vi "Day 7.vi"() -> ()   [LabVIEW 2023]
panel:
  out "Answer 2":i32
  out "Answer 1":i32
  out "used space":i32
  out "free space":i32
  out "sizes":i32[](array[numeric])
  out "paths":string[](array[string])
  in  "test":bool
  in  "test input":string="$ cd /\n$ ls\ndir a\n14848514 b.txt\n8504156 c.dat\ndir d\n$ cd a\n$ ls\ndir e\n29116 f\n2557 g\n62596 h.lst\n$ cd e\n$ ls\n584 i\n$ cd ..\n$ cd ..\n$ cd d\n$ ls\n4060174 j\n8033020 d.log\n5626152 d.ext\n7214296 k"
  in  "input":string="$ cd /\n$ ls\ndir csjncqmr\ndir fnfjhvsp\ndir mhfrct\ndir pgmgbfcl\ndir qcf\ndir wrsjr\n$ cd csjncqmr\n$ ls\n8827 vdrdm.pfj\n$ cd ..\n$ cd fnfjhvsp\n$ ls\ndir csjncqmr\ndir czpmg\n162385 dcgph\n7135 hff.cdt\n$ cd csjncqmr\n$ ls\n121543 gzjdsn.wlc\ndir ljq\n$ cd ljq\n$ ls\ndir cwlrlvf\ndir jpqjhhpg\n$ cd cwlrlvf\n$ ls\n151219 dcgph\n$ cd ..\n$ cd jpqjhhpg\n$ ls\n188355 dcgph\n38458 gfgl.hlg\n$ cd ..\n$ cd ..\n$ cd ..\n$ cd czpmg\n$ ls\n168232 dcgph\n143031 gzjdsn.wlc\n$ cd ..\n$ cd ..\n$ cd mhfrct\n$ ls\ndir clm\n66710 dcgph\n232576 mtfhpcnj\n$ cd clm\n$ ls\ndir pgmgbfcl\n$ cd pgmgbfcl\n$ ls\n110296 qbfhj.tmn\n$ cd ..\n$ cd ..\n$ cd ..\n$ cd pgmgbfcl\n$ ls\n163613 cgchl\ndir nnlr\n123977 rrwbnmlh.jtt\ndir tjhzggs\ndir wfl\n252837 wpgrl\n$ cd nnlr\n$ ls\n103051 flp\ndir qrhlzd\ndir rcgmhz\ndir snwrlr\ndir vgj\ndir znbzt\n$ cd qrhlzd\n$ ls\ndir crg\n246915 dcgph\n264791 fcphzfb.fmb\n299291 flp\ndir mjqsg\n297202 pgmgbfcl\ndir sbbzgbz\ndir wnsnssbg\n$ cd crg\n$ ls\n55556 flp\n185529 jswdvn\n$ cd ..\n$ cd mjqsg\n$ ls\ndir fnfjhvsp\ndir jfbzjz\ndir rwg\n$ cd fnfjhvsp\n$ ls\n24945 cctwbs\n170960 csjncqmr\n316168 ljffgvvz.zld\n187325 pgmgbfcl.fzv\n74133 qbfhj.tmn\ndir tjhzggs\ndir vjmgmdz\n$ cd tjhzggs\n$ ls\n287777 csjncqmr.nbd\n$ cd ..\n$ cd vjmgmdz\n$ ls\ndir vgpb\n$ cd vgpb\n$ ls\n202578 bbbg.hlr\n$ cd ..\n$ cd ..\n$ cd ..\n$ cd jfbzjz\n$ ls\n207736 tjhzggs.cql\n$ cd ..\n$ cd rwg\n$ ls\n184997 csjncqmr\n4378 dcgph\n55767 qnc.wvv\n$ cd ..\n$ cd ..\n$ cd sbbzgbz\n$ ls\n321376 csjncqmr\n317438 flp\n9263 hrs\n$ cd ..\n$ cd wnsnssbg\n$ ls\ndir jdjv\n$ cd jdjv\n$ ls\n153354 gzjdsn.wlc\n$ cd ..\n$ cd ..\n$ cd ..\n$ cd rcgmhz\n$ ls\ndir tjhzggs\n$ cd tjhzggs\n$ ls\n299192 jfbzjz.ttg\n$ cd ..\n$ cd ..\n$ cd snwrlr\n$ ls\n30314 csjncqmr.jvn\ndir hcf\n$ cd hcf\n$ ls\n81979 jfbzjz.pfz\n179459 ngh\n$ cd ..\n$ cd ..\n$ cd vgj\n$ ls\n278579 jbn.rgz\ndir jzj\ndir lnbhh\ndir pgmgbfcl\ndir qgvspcpm\n$ cd jzj\n$ ls\n295808 hrs\n220437 vqbcl\n$ cd ..\n$ cd lnbhh\n$ ls\n212203 nfmhd.hbq\n233853 qgz.mcd\n$ cd ..\n$ cd pgmgbfcl\n$ ls\ndir mmbdpj\n138462 mwcdrpm.spr\n288430 pgmgbfcl.pwd\n132880 rdmwtn.qjj\n41775 rfqb.djh\ndir rnd\n69597 thnbf\n$ cd mmbdpj\n$ ls\n158542 hrs\n306559 tjhzggs\n$ cd ..\n$ cd rnd\n$ ls\n223745 fnfjhvsp.hgt\n138236 gdmtnffs.cdm\ndir gmzb\ndir hvl\n266178 mzwmjl.rqq\ndir njpq\n33906 qbfhj.tmn\ndir tjhzggs\n$ cd gmzb\n$ ls\n186579 nsbfn.lsd\n$ cd ..\n$ cd hvl\n$ ls\n312925 csjncqmr.sbc\n75264 gqp\n81003 gzjdsn.wlc\n$ cd ..\n$ cd njpq\n$ ls\n188139 lbnrr.pwd\n213545 qgqddvwf.hfl\n$ cd ..\n$ cd tjhzggs\n$ ls\ndir dlwvc\n191782 jfbzjz\ndir tbldpln\n$ cd dlwvc\n$ ls\n75927 jvhjtnft\n260563 qbfhj.tmn\ndir vlg\n$ cd vlg\n$ ls\n187660 hgm\ndir rhr\n273019 tdgr.crr\n$ cd rhr\n$ ls\n286129 wnn.jgn\n$ cd ..\n$ cd ..\n$ cd ..\n$ cd tbldpln\n$ ls\n173546 pdfrsq.pnb\n$ cd ..\n$ cd ..\n$ cd ..\n$ cd ..\n$ cd qgvspcpm\n$ ls\ndir dhrbsl\n286566 fldhvbq\n209725 gzjdsn.wlc\n148148 nspz.gwc\n111003 tjhzggs\n$ cd dhrbsl\n$ ls\n58390 gzjdsn.wlc\n150545 hrs\n$ cd ..\n$ cd ..\n$ cd ..\n$ cd znbzt\n$ ls\n211651 gwhb.mfz\n$ cd ..\n$ cd ..\n$ cd tjhzggs\n$ ls\ndir hgr\n229076 jfbzjz.dfh\ndir ptfcbwwv\n51893 qbfhj.tmn\n97712 qgtvfh.hvs\n$ cd hgr\n$ ls\ndir hwvgjdq\ndir vwvbt\n$ cd hwvgjdq\n$ ls\ndir pgmgbfcl\n$ cd pgmgbfcl\n$ ls\ndir qgs\n$ cd qgs\n$ ls\n188108 hrs\n$ cd ..\n$ cd ..\n$ cd ..\n$ cd vwvbt\n$ ls\n169212 tfrm.gjb\n$ cd ..\n$ cd ..\n$ cd ptfcbwwv\n$ ls\n67829 lpszzl\n$ cd ..\n$ cd ..\n$ cd wfl\n$ ls\ndir hfcm\n$ cd hfcm\n$ ls\n73872 flp\n$ cd ..\n$ cd ..\n$ cd ..\n$ cd qcf\n$ ls\ndir ctjw\n177175 dwzmnpr\ndir fqldn\ndir hmjnnjjj\n301788 hrs\ndir lgmld\ndir pgmgbfcl\n76771 qzsbm.zdb\ndir scbgn\n234764 vhrlgcf\n$ cd ctjw\n$ ls\n139505 mflt.hnr\n$ cd ..\n$ cd fqldn\n$ ls\ndir bgq\n7260 flgrh.tmt\ndir fnfjhvsp\ndir fnr\ndir gsnqjmw\n10529 gzjdsn.wlc\n22877 hrs\ndir hzbrgrfq\ndir snmbwrzn\ndir tjhzggs\n6773 tzhsjsc\n$ cd bgq\n$ ls\n40780 gzjdsn.wlc\n233301 mnzdbpc\ndir mpdjgbgf\n303076 qbfhj.tmn\ndir qjs\n189723 sbzn.dtj\ndir vhnqcrd\n$ cd mpdjgbgf\n$ ls\n227105 dcgph\n298219 dprcwts.vdt\n$ cd ..\n$ cd qjs\n$ ls\n214072 pgmgbfcl\n264897 qbfhj.tmn\n$ cd ..\n$ cd vhnqcrd\n$ ls\n178950 fnfjhvsp\n180561 pgmgbfcl.mst\n312980 pgmgbfcl.twp\n$ cd ..\n$ cd ..\n$ cd fnfjhvsp\n$ ls\n141191 fnfjhvsp.bng\n81709 pgmgbfcl.sfw\n$ cd ..\n$ cd fnr\n$ ls\n316638 flp\ndir fnfjhvsp\ndir fqdnn\n267054 gdnln\ndir hfcrzwvm\ndir rdljd\n319112 wpcmfbr.zgp\n$ cd fnfjhvsp\n$ ls\n115581 hrs\ndir jfbzjz\n$ cd jfbzjz\n$ ls\n170398 qbfhj.tmn\n$ cd ..\n$ cd ..\n$ cd fqdnn\n$ ls\ndir cfg\ndir jbjltw\n$ cd cfg\n$ ls\ndir qljztr\ndir tnsw\ndir zhnqp\n$ cd qljztr\n$ ls\n64638 bnlsrfb\n63440 csjncqmr\n206111 gzjdsn.wlc\n207890 hrs\n265995 pgmgbfcl.zcw\n$ cd ..\n$ cd tnsw\n$ ls\n85166 lsflqzmc\n$ cd ..\n$ cd zhnqp\n$ ls\n217666 csjncqmr.cch\n$ cd ..\n$ cd ..\n$ cd jbjltw\n$ ls\n88043 dcgph\n238483 hrs\n189734 jnvwjs\n243936 pgmgbfcl.wsr\n$ cd ..\n$ cd ..\n$ cd hfcrzwvm\n$ ls\ndir vwc\n$ cd vwc\n$ ls\n82566 shc.qhj\n$ cd ..\n$ cd ..\n$ cd rdljd\n$ ls\n68011 ptw.bgd\n$ cd ..\n$ cd ..\n$ cd gsnqjmw\n$ ls\n236818 gzjdsn.wlc\n$ cd ..\n$ cd hzbrgrfq\n$ ls\n240924 dcgph\ndir dcjsv\ndir dsrzdjfm\ndir fnfjhvsp\ndir hnzm\ndir mqb\n94014 smpnth.bbm\n$ cd dcjsv\n$ ls\n316708 cmddvb\ndir fnfjhvsp\n$ cd fnfjhvsp\n$ ls\ndir fnfjhvsp\n$ cd fnfjhvsp\n$ ls\ndir jqlcvds\n$ cd jqlcvds\n$ ls\n51018 dqfbq.ggm\n$ cd ..\n$ cd ..\n$ cd ..\n$ cd ..\n$ cd dsrzdjfm\n$ ls\n262938 csjncqmr.dmm\n125129 mwcnlvhv.szp\n150590 qbfhj.tmn\ndir rrrzpsn\n196430 vbdgb\ndir vsfbwfdl\n$ cd rrrzpsn\n$ ls\ndir tjhzggs\n281655 tjhzggs.btg\ndir tsjzf\n$ cd tjhzggs\n$ ls\n291402 gbl\ndir hctmr\ndir hqdmpwl\n225075 hrs\ndir jfbzjz\n51032 tjhzggs.qzr\n$ cd hctmr\n$ ls\n113430 qbfhj.tmn\n$ cd ..\n$ cd hqdmpwl\n$ ls\n67634 tjhzggs\n$ cd ..\n$ cd jfbzjz\n$ ls\n193552 nmvl.tzj\n197076 pgmgbfcl\n11047 tjhzggs\n$ cd ..\n$ cd ..\n$ cd tsjzf\n$ ls\n36205 jwmdtdjv\n$ cd ..\n$ cd ..\n$ cd vsfbwfdl\n$ ls\n288660 flp\n185921 jfbzjz\ndir mqmvtddt\n124423 nfbfq.dln\ndir wzbc\n$ cd mqmvtddt\n$ ls\n85529 bhjp.vvj\n$ cd ..\n$ cd wzbc\n$ ls\n77316 flp\n271730 pgmgbfcl.lcd\n$ cd ..\n$ cd ..\n$ cd ..\n$ cd fnfjhvsp\n$ ls\n47666 mpwtvwd.fwr\n$ cd ..\n$ cd hnzm\n$ ls\n157672 flp\n294957 gzjdsn.wlc\n297187 lbssg\n24223 qbfhj.tmn\ndir rdnqrgt\n177449 tld.tsd\n$ cd rdnqrgt\n$ ls\ndir nltjzrrr\n217347 vrb.gcd\n$ cd nltjzrrr\n$ ls\ndir zzd\n$ cd zzd\n$ ls\n47464 flp\ndir fnfjhvsp\n$ cd fnfjhvsp\n$ ls\n89424 qtzfddz.btd\n$ cd ..\n$ cd ..\n$ cd ..\n$ cd ..\n$ cd ..\n$ cd mqb\n$ ls\n105537 tjhzggs.wns\n$ cd ..\n$ cd ..\n$ cd snmbwrzn\n$ ls\ndir mqt\ndir nsdrn\ndir rjn\n$ cd mqt\n$ ls\n233842 pgmgbfcl\n$ cd ..\n$ cd nsdrn\n$ ls\n67018 dcgph\n17296 flp\n274166 gzjdsn.wlc\n186308 jfbzjz\n280195 lvbsrvwm.zlq\ndir pjv\ndir thlp\n$ cd pjv\n$ ls\n123190 rfbj.gmq\n$ cd ..\n$ cd thlp\n$ ls\n141308 flp\n188164 jfbzjz\n299013 pgmgbfcl\n171259 qbfhj.tmn\ndir qsljb\n$ cd qsljb\n$ ls\n291980 glcnlj.swh\n$ cd ..\n$ cd ..\n$ cd ..\n$ cd rjn\n$ ls\n181047 fqmhpg.hpl\n$ cd ..\n$ cd ..\n$ cd tjhzggs\n$ ls\ndir csjncqmr\n274202 fhfjvdjc.swt\ndir fnfjhvsp\n97050 frbpp.wch\ndir gnbtgdr\ndir jfbzjz\ndir lpg\ndir pgmgbfcl\ndir twcdfdcv\ndir wzd\ndir zllcflrn\n$ cd csjncqmr\n$ ls\ndir chpmwsfj\ndir csjncqmr\n57088 fnfjhvsp.jqg\n52097 vgcm.dpv\n$ cd chpmwsfj\n$ ls\n279480 tjhzggs.srw\n$ cd ..\n$ cd csjncqmr\n$ ls\n13716 dcgph\ndir fqb\ndir jfbzjz\ndir msvlnt\n88312 pgmgbfcl.qcf\n$ cd fqb\n$ ls\ndir mmjfbvq\n$ cd mmjfbvq\n$ ls\n79822 flp\n$ cd ..\n$ cd ..\n$ cd jfbzjz\n$ ls\n302531 csjncqmr\n164326 dcgph\n8277 fnfjhvsp.rbv\ndir jgsrgrtc\ndir zwdgcd\n$ cd jgsrgrtc\n$ ls\n60317 gzjdsn.wlc\n$ cd ..\n$ cd zwdgcd\n$ ls\n171967 fpls.fvd\n$ cd ..\n$ cd ..\n$ cd msvlnt\n$ ls\n83178 cnhzh\n11226 tjhzggs\n$ cd ..\n$ cd ..\n$ cd ..\n$ cd fnfjhvsp\n$ ls\n89882 dcgph\n212817 qbfhj.tmn\n257899 tjhzggs\n$ cd ..\n$ cd gnbtgdr\n$ ls\ndir flltghn\ndir fnfjhvsp\ndir jfbzjz\n300698 ngcsnwb\n292809 qtcqhdq\ndir vbwjgf\n280270 wbzcr.sgn\n$ cd flltghn\n$ ls\n111452 rhgfv\n$ cd ..\n$ cd fnfjhvsp\n$ ls\ndir lbznfb\n31273 nrtrqqc.cth\n$ cd lbznfb\n$ ls\n175736 ljpr.cwm\n$ cd ..\n$ cd ..\n$ cd jfbzjz\n$ ls\n237625 tjhzggs\n$ cd ..\n$ cd vbwjgf\n$ ls\n269242 jrrw.ljb\n106705 pqnbrbt\n$ cd ..\n$ cd ..\n$ cd jfbzjz\n$ ls\ndir dnn\n$ cd dnn\n$ ls\n19045 dcgph\n187257 tjhzggs.qzg\n$ cd ..\n$ cd ..\n$ cd lpg\n$ ls\n101509 fnfjhvsp.nnt\n221211 ldgjngjq\n$ cd ..\n$ cd pgmgbfcl\n$ ls\ndir bzbdphz\n37920 flp\ndir wpsm\n$ cd bzbdphz\n$ ls\n252099 ffsfqfdw\n312106 htft\n298880 jfbvz.znw\n135204 lrwccthr\ndir zhbqf\n108144 zsbbfhz.drr\n$ cd zhbqf\n$ ls\ndir gtw\n298022 svpgsrgj.ljz\n$ cd gtw\n$ ls\ndir csjncqmr\ndir rpzjg\n$ cd csjncqmr\n$ ls\n278962 flp\n272127 tjhzggs\n$ cd ..\n$ cd rpzjg\n$ ls\n92241 flp\n$ cd ..\n$ cd ..\n$ cd ..\n$ cd ..\n$ cd wpsm\n$ ls\n15936 flp\n241514 qbfhj.tmn\n245049 rjgwzlq.qrw\n$ cd ..\n$ cd ..\n$ cd twcdfdcv\n$ ls\n140758 bjm\n78772 dcgph\n114059 mqsgrc.qcb\n$ cd ..\n$ cd wzd\n$ ls\ndir fnfjhvsp\ndir mcbnp\n$ cd fnfjhvsp\n$ ls\n72702 csjncqmr.jfn\n120586 dcgph\n$ cd ..\n$ cd mcbnp\n$ ls\n12494 fnfjhvsp.frc\n182092 gsv\n17859 pdbvmblc.vng\n116984 pfbdf\n113843 prshrmg.srm\n$ cd ..\n$ cd ..\n$ cd zllcflrn\n$ ls\n30966 flp\n245820 jfbzjz.rnd\n$ cd ..\n$ cd ..\n$ cd ..\n$ cd hmjnnjjj\n$ ls\n134366 dcgph\n212399 dtsb\n255795 zhbcjtr\n$ cd ..\n$ cd lgmld\n$ ls\n55248 pgmgbfcl\n62265 pgmgbfcl.nbg\n240733 zhmff\n$ cd ..\n$ cd pgmgbfcl\n$ ls\n232717 fnfjhvsp\n219581 gtcjbwpz.lmz\n47399 gzjdsn.wlc\n22814 hjqf\n296672 hrs\ndir nrzf\ndir wqgcmnpp\ndir wwvmdjz\ndir zlhv\n$ cd nrzf\n$ ls\n18406 dcgph\ndir mhm\n$ cd mhm\n$ ls\n95168 pgmgbfcl.hqv\n$ cd ..\n$ cd ..\n$ cd wqgcmnpp\n$ ls\ndir csjncqmr\n189963 dvcd.tnh\ndir gzqrt\ndir njffft\ndir qvqp\n6981 tjhzggs\ndir wgfnlfsd\n$ cd csjncqmr\n$ ls\n307371 cdptrw.rfm\n$ cd ..\n$ cd gzqrt\n$ ls\ndir pwsqss\n$ cd pwsqss\n$ ls\n173397 flp\n$ cd ..\n$ cd ..\n$ cd njffft\n$ ls\ndir bzhzg\ndir tjhzggs\n$ cd bzhzg\n$ ls\n213821 pgmgbfcl\n$ cd ..\n$ cd tjhzggs\n$ ls\ndir szvfzgj\n$ cd szvfzgj\n$ ls\n196306 tjhzggs.hjh\n$ cd ..\n$ cd ..\n$ cd ..\n$ cd qvqp\n$ ls\ndir pgmgbfcl\n$ cd pgmgbfcl\n$ ls\n114456 flp\n252954 pgmgbfcl\n$ cd ..\n$ cd ..\n$ cd wgfnlfsd\n$ ls\n212011 gzjdsn.wlc\n$ cd ..\n$ cd ..\n$ cd wwvmdjz\n$ ls\n70022 dcgph\ndir hjgvstp\ndir jhgb\n276853 qbfhj.tmn\n242756 qdqswjjd.wnn\ndir tjhzggs\n292963 wcgmgmz.shb\n$ cd hjgvstp\n$ ls\n24056 tdjwdw\n$ cd ..\n$ cd jhgb\n$ ls\n90571 gzjdsn.wlc\n132326 rrvfml.dms\n$ cd ..\n$ cd tjhzggs\n$ ls\n29139 dmrsz.qhc\n$ cd ..\n$ cd ..\n$ cd zlhv\n$ ls\n315120 dcgph\n290175 pgvlcvpb\n$ cd ..\n$ cd ..\n$ cd scbgn\n$ ls\n258300 bcchv.qsn\n$ cd ..\n$ cd ..\n$ cd wrsjr\n$ ls\ndir csjncqmr\ndir jfbzjz\ndir nmfmqb\ndir svgtrz\ndir zjvhmd\n$ cd csjncqmr\n$ ls\n148619 qbfhj.tmn\n$ cd ..\n$ cd jfbzjz\n$ ls\ndir csjncqmr\ndir flrhpzt\ndir fnfjhvsp\ndir gpwv\ndir lwrtc\n$ cd csjncqmr\n$ ls\ndir czmlfmf\n137365 flp\ndir hggbs\n107369 mpgm.lbl\n$ cd czmlfmf\n$ ls\ndir hnpjvq\n$ cd hnpjvq\n$ ls\n41339 fnfjhvsp.wnv\n$ cd ..\n$ cd ..\n$ cd hggbs\n$ ls\n273367 qbfhj.tmn\n$ cd ..\n$ cd ..\n$ cd flrhpzt\n$ ls\n200923 fwb\n62059 hrs\n$ cd ..\n$ cd fnfjhvsp\n$ ls\ndir gdnmpgn\n256037 hrs\n$ cd gdnmpgn\n$ ls\n64024 jmww.gbb\n$ cd ..\n$ cd ..\n$ cd gpwv\n$ ls\n159155 hrs\n$ cd ..\n$ cd lwrtc\n$ ls\n150299 nzvqj.dsv\n129702 pgmgbfcl.lrt\ndir zvgb\n$ cd zvgb\n$ ls\n304137 hrs\n$ cd ..\n$ cd ..\n$ cd ..\n$ cd nmfmqb\n$ ls\n139823 jfbzjz\n299946 nqqscdn.wsw\n$ cd ..\n$ cd svgtrz\n$ ls\ndir jdlvtm\n123801 phhrgrbs\n$ cd jdlvtm\n$ ls\n267972 tbgcnf.pqz\n$ cd ..\n$ cd ..\n$ cd zjvhmd\n$ ls\n287427 csjncqmr.tfj\n297578 hhhp.jvt\n"
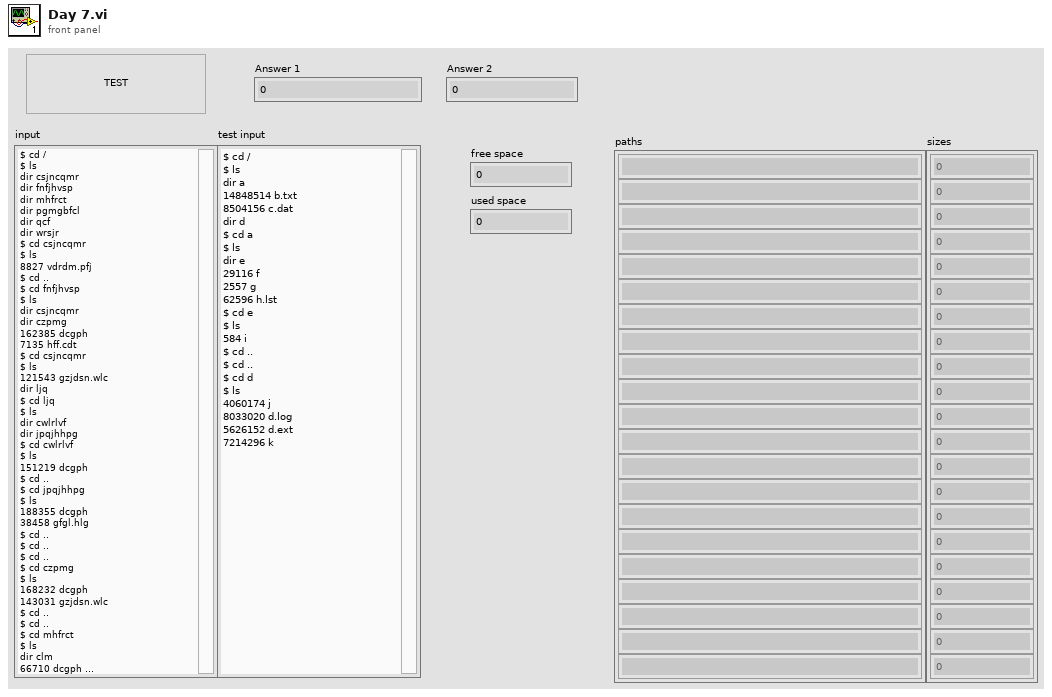
[diagram p1: front panel]
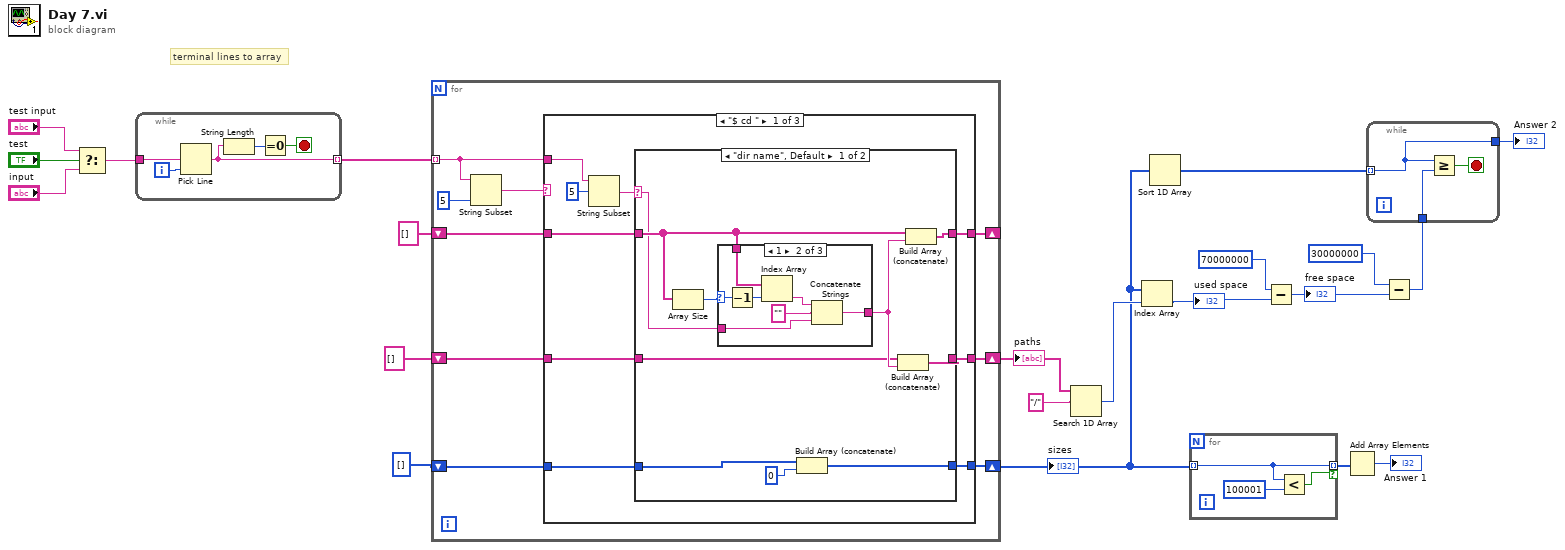
[diagram p0: block diagram]
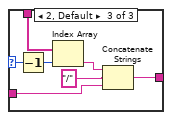
[diagram p3: hidden frame]
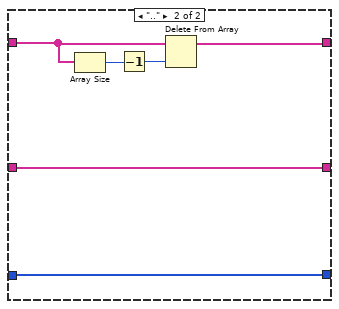
[diagram p4: hidden frame]
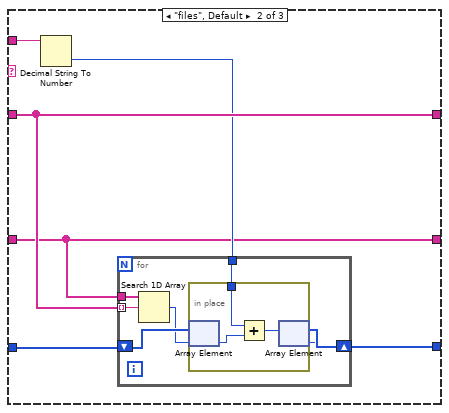
[diagram p5: hidden frame]
diagram:
  # "terminal lines to array"
  n1 = Select(t="test input", s="test", f="input") -> (s? t:f=w20:string)
  n2 = while {
    tunnel: w20 -> [w23]
    tunnel: [w22] -> w17 mode=indexing
    i -> [w24]
    stop <- w25 stop-if-true
    n3 = Pick Line(multi-line string=w23, line index=w24) -> (output string=w22:string)  [unwired: 1 in]
    n4 = String Length(string=w22) -> (length=w26:i32)
    n5 = Equal To 0?(x=w26) -> (x = 0?=w25:bool)
  }
  n6 = for {
    tunnel: w17 -> [w33] mode=indexing
    shift-right: [w32] -> _
    shift-left: string[] [] -> [w31]
    shift-right: [w28] -> w4
    shift-left: i32[] [] -> [w27]
    shift-right: [w30] -> w15
    shift-left: string[] [] -> [w29]
    n7 = String Subset(string=w33, length (rest)=5 ("length (rest)")) -> (substring=w34:string)  [unwired: 1 in]
    n8 = case shown="\"$ cd \"" w34 {
      tunnel: w33 -> [w44 w81 _]
      tunnel: [w41 w80 w93] -> w32
      tunnel: w31 -> [w40 w80 w93]
      tunnel: [w39 w76 w92] -> w30
      tunnel: w29 -> [w38 w76 w92]
      tunnel: [w37 w78 w91] -> w28
      tunnel: w27 -> [w36 w79 w91]
      frame "$ cd " {
        n9 = String Subset(string=w44, offset (0)=5 ("length (rest)")) -> (substring=w42:string)  [unwired: 1 in]
        n10 = case shown="\"dir name\", Default" w42 {
          selector: w42 -> [w52 _]
          tunnel: [w54 w75] -> w41
          tunnel: w40 -> [w53 w74]
          tunnel: [w49 w71] -> w39
          tunnel: w38 -> [w48 w71]
          tunnel: [w47 w70] -> w37
          tunnel: w36 -> [w46 w70]
          frame "dir name", Default {
            n11 = Array Size(array=w53) -> (size(s)=w51:i32)
            n12 = case shown="1" w51 {
              selector: w51 -> [_ w57 w64]
              tunnel: w53 -> [_ w62 w69]
              tunnel: w52 -> [w55 w59 w66]
              tunnel: [w55 w58 w65] -> w50
              frame 0 {
              }
              frame 1 {
                n13 = Decrement(x=w57) -> (x-1=w56:i32)
                n14 = Index Array(array=w62, index=w56) -> (element=w61:string)
                n15 = Concatenate Strings(w61, "" ("string"), w59) -> (w58:string)
              }
              frame 2, Default {
                n16 = Decrement(x=w64) -> (x-1=w63:i32)
                n17 = Index Array(array=w69, index=w63) -> (element=w68:string)
                n18 = Concatenate Strings(w68, "/" ("string"), w66) -> (w65:string)
              }
            }
            n19 = Build Array (concatenate)(w46, 0) -> (w47:i32[])
            n20 = Build Array (concatenate)(w48, w50) -> (w49:string[])
            n21 = Build Array (concatenate)(w53, w50) -> (w54:string[])
          }
          frame ".." {
            n22 = Array Size(array=w74) -> (size(s)=w73:i32)
            n23 = Decrement(x=w73) -> (x-1=w72:i32)
            n24 = Delete From Array(array=w74, index=w72) -> (array with subset deleted=w75:string[])  [unwired: 1 in, 1 out]
          }
        }
      }
      frame "files", Default {
        n25 = Decimal String To Number(string=w81) -> (number=w77:i32)  [unwired: 2 in, 1 out]
        n26 = for {
          tunnel: w80 -> [w86] mode=indexing
          tunnel: w76 -> [w87]
          shift-right: [w83] -> w78
          shift-left: w79 -> [w85]
          tunnel: w77 -> [w82]
          n27 = Search 1D Array(1D array=w87, element=w86) -> (index of element=w84:i32)  [unwired: 1 in]
          n28 = in-place {
            in-place-border: w82 -> [w88]
            n29 = in-place-array #1(w85, w84) -> (w90:i32)
            n30 = Add(x=w88, y=w90) -> (x+y=w89:i32)
            n31 = in-place-array #1(w89) -> (w83:i32[])  [unwired: 1 out]
          }
        }
      }
      frame "$ ls", "dir " {
      }
    }
  }
  "paths" <- w15
  "sizes" <- w4
  n32 = Search 1D Array(1D array=w15, element="/") -> (index of element=w13:i32)  [unwired: 1 in]
  n33 = Index Array(array=w4, index=w13) -> (element=w8:i32)
  "used space" <- w8
  n34 = Sort 1D Array(array=w4) -> (sorted array=w1:i32[])
  n35 = for {
    tunnel: w4 -> [w95] mode=indexing
    tunnel: [w95] -> w6 mode=indexing if=w94
    n36 = Less?(x=w95, y=100001) -> (x < y?=w94:bool)
  }
  n37 = Subtract(x=70000000 ("max value 2"), y=w8) -> (x-y=w9:i32)
  "free space" <- w9
  n38 = Add Array Elements(numeric array=w6) -> (sum=→"Answer 1":i32)
  n39 = Subtract(x=30000000 ("max value 2"), y=w9) -> (x-y=w3:i32)
  n40 = while {
    tunnel: w1 -> [w97] mode=indexing
    tunnel: w3 -> [w99]
    tunnel: [w97] -> w2
    stop <- w98 stop-if-true
    n41 = Greater Or Equal?(x=w97, y=w99) -> (x >= y?=w98:bool)
  }
  "Answer 2" <- w2
